vi "Lockin.Low Pass Filter (subVI).vi"(8 "error in (no error)":errorcluster, 9 "Element Data":i32, 10 "signal in":waveform(dbl)[](array[waveform]), 11 "Lockin.DAQ in":refnum<class "Instrument.DAQ.lvclass">) -> (0 "error out":errorcluster, 1 "Fc (Hz)":dbl, 2 "signal out":waveform(dbl)[](array[waveform]))   [LabVIEW 2019, in "DSP.lvclass"]
uses:
  DSP.lvclass
  Instrument.DAQ/Instrument.DAQ.lvclass
  C:/Program Files (x86)/National Instruments/LabVIEW 2019/vi.lib/JKI/JKI SMO/SMO/SMO.lvclass
panel:
  out "Lockin.DAQ out":refnum<class "Instrument.DAQ.lvclass">
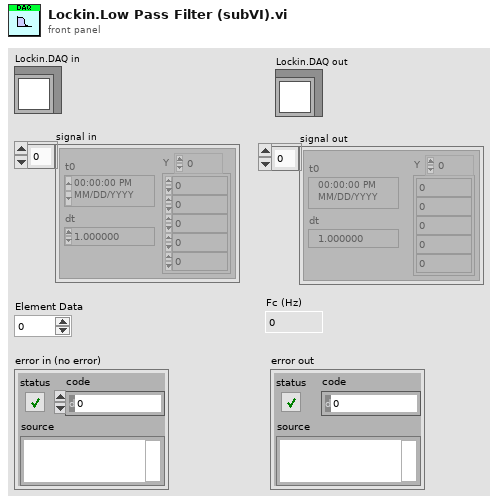
[diagram p1: front panel]
types:
  T1 = typedef "NI_DigFilterLicensed.lvlib/DFD Filter Obj.ctl" = cluster{"mSRate_Fs":dbl, "mSRate_Version":string, "mSRate_Comments":string, "mSRate_OrgCoef":T2, "mSRate_CurCoef":T2, "mSRate_Quantized?":bool, "mSRate_QCoef":T2, "mSRate_QSettings":T4[], "mSRate_Order":i32, "mSRate_Scaling":cluster{"mSRate_ScaleByPowerOf2?":bool, "mSRate_ScaleType":T6}}
  T2 = typedef "NI_DigFilterLicensed.lvlib/DFD Filter Coef.ctl" = cluster{"type":T3, "gain":dbl, "coef a (k)":dbl[], "coef b (v)":dbl[]}
  T3 = typedef "NI_DigFilterLicensed.lvlib/DFD Filter Structure Type Selector.ctl" = enum16{"Undefined", "FIR Direct Form", "FIR Direct Form Transposed", "FIR Symmetric", "FIR Antisymmetric", "IIR Direct Form I", "IIR Direct Form I Transposed", "IIR Direct Form II", "IIR Direct Form II Transposed", "IIR Cascaded Second Order Sections Form I", "IIR Cascaded Second Order Sections Form I Transposed", "IIR Cascaded Second Order Sections Form II", "IIR Cascaded Second Order Sections Form II Transposed", "Lattice Allpass (basic sections)", "Lattice Allpass (one multiplier sections)", "Lattice Allpass (normalized sections)", "Lattice AR (basic sections)", "Lattice AR (one multiplier sections)", "Lattice AR (normalized sections)", "Lattice MA (minimum phase)", "Lattice MA (maximum phase)", "Lattice ARMA (basic sections)", "Lattice ARMA (one multiplier sections)", "Lattice ARMA (normalized sections)"}
  T4 = typedef "NI_DigFilterLicensed.lvlib/dfd_Internal Quantization Settings.ctl" = cluster{"source":T5, "wl":i16, "iwl":i16, "overflow mode":enum16{"Saturation", "Wrap"}, "rounding mode":enum16{"Nearest", "Truncation"}, "signed?":bool}
  T5 = typedef "NI_DigFilterLicensed.lvlib/dfd_Internal Quantization Srcs.ctl" = u16
  T6 = typedef "NI_DigFilterLicensed.lvlib/DFD Coef Norm Type.ctl" = enum16{"No Norm", "Time Domain 1-Norm", "Time Domain 2-Norm", "Time Domain Inf-Norm"}
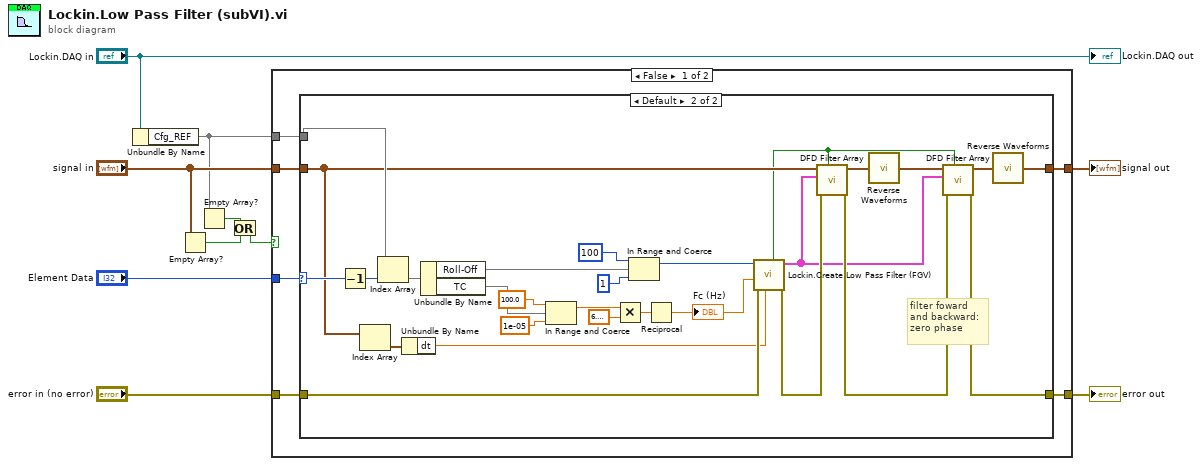
[diagram p0: block diagram]
diagram:
  n1 = Unbundle By Name("Lockin.DAQ in") -> ("Cfg_REF"=w4)
  n2 = Empty Array?(array="signal in") -> (empty?=w2:bool)
  n3 = Empty Array?(array=w4) -> (empty?=w3:bool)
  n4 = Or(x=w3, y=w2) -> (x .or. y?=w1:bool)
  n5 = case shown="False" w1 {
    tunnel: "error in (no error)" -> [w16 w48]
    tunnel: [w15 w48] -> w9
    tunnel: [w14 w47] -> w8
    tunnel: "Element Data" -> [w12 _]
    tunnel: "signal in" -> [w13 w47]
    tunnel: w4 -> [w11 _]
    frame False {
      n6 = case shown="Default" w12 {
        selector: w12 -> [_ w36]
        tunnel: w16 -> [w18 w26]
        tunnel: [w18 w28] -> w15
        tunnel: w13 -> [w17 w33]
        tunnel: [w17 w29] -> w14
        tunnel: w11 -> [_ w34]
        frame 0 {
        }
        frame Default {
          # "filter foward\nand backward:\nzero phase"
          n7 = Decrement(x=w36) -> (x-1=w35:i32)
          n8 = Index Array(array=w33) -> (element=w46:waveform(dbl))  [unwired: 1 in]
          n9 = Index Array(array=w34, index=w35) -> (element=w45)
          n10 = Unbundle By Name(w46) -> ("dt"=w22:dbl)
          n11 = Unbundle By Name(w45) -> ("Roll-Off"=w19, "TC"=w44)
          n12 = In Range and Coerce(upper limit=100.0, x=w44, lower limit=1e-05) -> (coerced(x)=w37:dbl)  [unwired: 1 out]
          n13 = Multiply(x=w37, y=6.283185307179586) -> (x*y=w41:dbl)
          n14 = In Range and Coerce(upper limit=100, x=w19, lower limit=1) -> (coerced(x)=w25:i32)  [unwired: 1 out]
          n15 = Reciprocal(x=w41) -> (1/x=w23:dbl)
          "Fc (Hz)" <- w23
          n16 = call "Lockin.Create Low Pass Filter (FGV).vi"("fs (Hz)"=w22, "error in (no error)"=w26, "Low Pass Cutoff (Hz)"=w23, "order"=w25) -> ("error out"=w24:errorcluster, "Filters out"=w20:T1[], "init out"=w21:bool)  [unwired: 5 in]
          n17 = call "DFD Filter Array.vi"("init (F)"=w21, "error in (no error)"=w24, "filters"=w20, "signal in"=w33) -> ("error out"=w27:errorcluster, "signal out"=w30:waveform(dbl)[])  [unwired: 6 in]
          n18 = call "Reverse Waveforms.vi"("signal in"=w30) -> ("Array"=w32:waveform(dbl)[])
          n19 = call "DFD Filter Array.vi"("init (F)"=w21, "error in (no error)"=w27, "filters"=w20, "signal in"=w32) -> ("error out"=w28:errorcluster, "signal out"=w31:waveform(dbl)[])  [unwired: 6 in]
          n20 = call "Reverse Waveforms.vi"("signal in"=w31) -> ("Array"=w29:waveform(dbl)[])
        }
      }
    }
    frame True {
    }
  }
  "error out" <- w9
  "signal out" <- w8
  "Lockin.DAQ out" <- "Lockin.DAQ in"
